vi "Cylinder To Actuator.vi"(8 "error in (no error)":errorcluster, 9 "FC2 Measured Value":dbl format="%.3f", 10 "FC1 Measured Value":dbl format="%.3f", 11 "Cylinder To Actuator Forces in":refnum<class "Cylinder To Actuator Forces.lvclass">) -> (0 "error out":errorcluster, 1 "Lateral Force":dbl format="%.3f", 2 "Axial Force":dbl format="%.3f", 3 "Cylinder To Actuator Forces out":refnum<class "Cylinder To Actuator Forces.lvclass">)   [LabVIEW 2015, in "Cylinder To Actuator Forces.lvclass"]
uses:
  Cylinder To Actuator Forces.lvclass
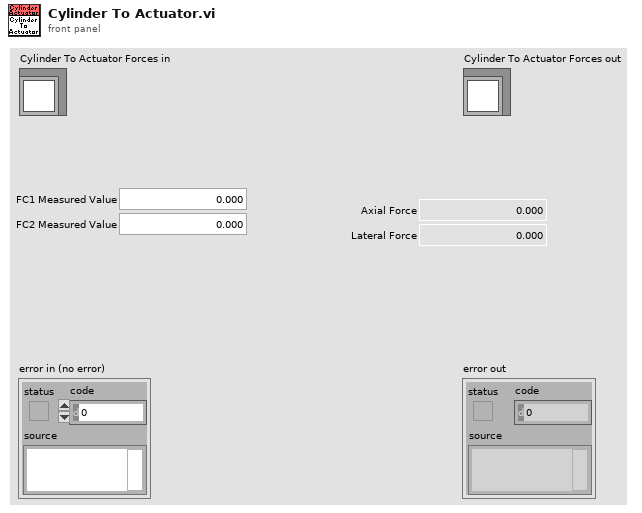
[diagram p1: front panel]
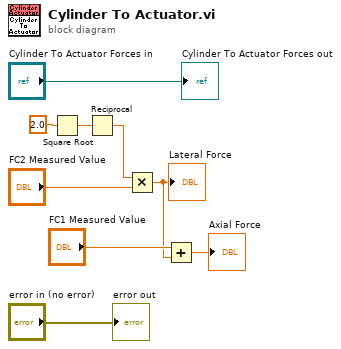
[diagram p0: block diagram]
diagram:
  n1 = Square Root(x=2.0) -> (sqrt(x)=w6:dbl)
  n2 = Reciprocal(x=w6) -> (1/x=w4:dbl)
  n3 = Multiply(x=w4, y="FC2 Measured Value") -> (x*y=w2:dbl)
  "Lateral Force" <- w2
  n4 = Add(x="FC1 Measured Value", y=w2) -> (x+y=→"Axial Force":dbl)
  "error out" <- "error in (no error)"
  "Cylinder To Actuator Forces out" <- "Cylinder To Actuator Forces in"
